vi "定时器更新溢出中断实验.vi"   [LabVIEW 2011]
uses:
  <vilib>/STM32_DriverVI_Interface_F4/Timer/TIMX Interrupt_F4.ctl
  <vilib>/STM32_DriverVI_Interface/Interrupt/PreemptionPriority_0.ctl
  <vilib>/STM32_DriverVI_Interface/Interrupt/SubPriority_0.ctl
  <vilib>/STM32_DriverVI_Interface_F4/Timer/TIM2_Int_Channel_F4.ctl
  <vilib>/STM32_DriverVI_Interface_F4/Timer/TIM2_Flag_F4.ctl
  <vilib>/STM32_DriverVI_Interface_F4/Timer/Reload Mode_F4.ctl
  <vilib>/STM32_DriverVI_Interface_F4/Timer/TIM2 Init_F4.vi
  <vilib>/STM32_DriverVI_Interface_F4/Timer/TIM Priority Set_0_F4.vi
  <vilib>/STM32_DriverVI_Interface_F4/Timer/TIM2 SW Interrupt_F4.vi
  <vilib>/STM32_DriverVI_Interface_F4/Timer/Clear_TIM2_Flag_F4.vi
  <vilib>/STM32_DriverVI_Interface_F4/Timer/TIM2 Int Permit_UnPermit_F4.vi
  <vilib>/STM32_DriverVI_Interface_F4/Timer/TIM2 Int Enable_Disable_F4.vi
  <vilib>/STM32_DriverVI_Interface_F4/Timer/TIM2 Update Interval_F4.vi
types:
  T1 = typedef "TIM2_Flag_F4.ctl" = enum8{"TIM2_Update(Overflow)", "TIM2_Channel_1", "TIM2_Channel_2", "TIM2_Channel_3", "TIM2_Channel_4", "TIM2_Reserved……", "TIM2_Trigger（Pulse）"}
  T2 = typedef "中断使能禁止.ctl" = enum8{"Disable", "Enable"}
  T3 = typedef "允许或禁止TIM中断_F4.ctl" = enum8{"禁止", "允许"}
  T4 = typedef "TIM2_Int_Channel_F4.ctl" = enum8{"TIM2_Update(Overflow)", "TIM2_Channel_1", "TIM2_Channel_2", "TIM2_Channel_3", "TIM2_Channel_4", "TIM2_Reserved……", "TIM2_Trigger（Pulse）"}
  T5 = typedef "SubPriority_0.ctl" = enum8{"Priority_0（High）", "Priority_1", "Priority_2", "Priority_3", "Priority_4", "Priority_5", "Priority_6", "Priority_7", "Priority_8", "Priority_9", "Priority_10", "Priority_11", "Priority_12", "Priority_13", "Priority_14", "Priority_15（Low）"}
  T6 = typedef "PreemptionPriority_0.ctl" = enum8{"Priority_0（Only）"}
  T7 = typedef "TIMX Interrupt_F4.ctl" = u8
  T8 = typedef "TIMX计数时钟频率_F4.ctl" = u16
  T9 = typedef "Reload Mode_F4.ctl" = enum8{"写入时立刻重载", "发生更新中断时重载"}
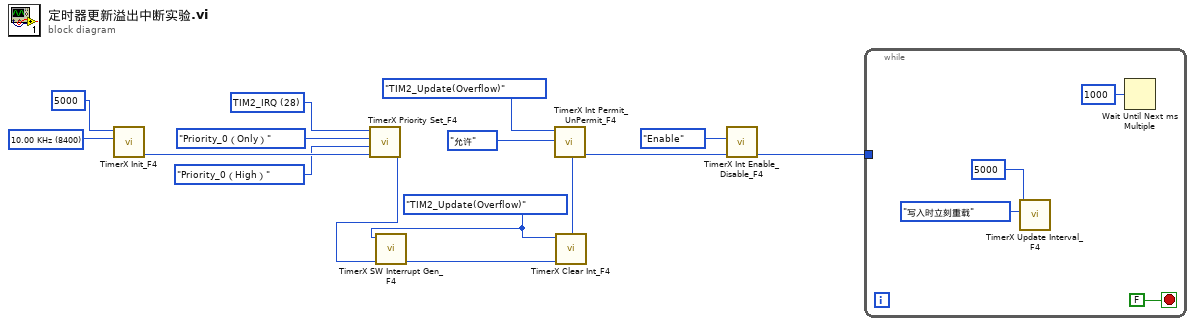
[diagram p0: block diagram]
diagram:
  w1 = TIM2_Flag_F4."TIM2_Update(Overflow)" ("TIM2_Flag")
  w13 = T7 28 items=["WWDG_IRQ"=0, "RTC_WKUP_IRQ"=3, "RTC_Alarm_IRQ"=41, "TIM1_BRK_TIM9_IRQ"=24, "TIM1_UP_TIM10_IRQ"=25, "TIM1_TRG_COM_TIM11_IRQ"=26, "TIM1_CC_IRQ"=27, "TIM2_IRQ"=28, "TIM3_IRQ"=29, "TIM4_IRQ"=30, "TIM5_IRQ"=50, "TIM6_IRQ"=54, "TIM7_IRQ"=55, "TIM8_BRK_TIM12_IRQ"=43, "TIM8_UP_TIM13_IRQ"=44, "TIM8_TRG_COM_TIM14_IRQ"=45, "TIM8_CC_IRQ"=46] ("IO 中断号设置")
  w14 = T8 8400 items=["84.00 MHz"=1, "42.00 MHz"=2, "28.00 MHz"=3, "21.00 MHz"=4, "12.000 MHz"=7, "7.000 MHz"=12, "4.000 MHz"=21, "1.000 MHz"=84, "-------------"=0, "500.0 KHz"=168, "250.0 KHz"=336, "100.0 KHz"=840, "50.00 KHz"=1680, "10.00 KHz"=8400] ("时钟预分频数")
  n1 = call-poly <vilib>:"TimerX Init_F4.vi"("时钟预分频数"=w14, "自动重装值"=u16 5000) -> ("err_out"=w12:u8)  [unwired: 9 in]
  n2 = call-poly <vilib>:"TimerX Priority Set_F4.vi"("err_in"=w12, "响应优先级"=SubPriority_0."Priority_0（High）", "抢占优先级"=PreemptionPriority_0."Priority_0（Only）", "TIM 中断号设置"=w13) -> ("err_out"=w3:u8)  [unwired: 6 in, 1 out]
  n3 = call-poly <vilib>:"TimerX SW Interrupt Gen_F4.vi"("err_in"=w3, "TIM2_Flag"=w1) -> ("err_out"=w4:u8)  [unwired: 9 in]
  n4 = call-poly <vilib>:"TimerX Clear Int_F4.vi"("err_in"=w4, "TIM2_Flag"=w1) -> ("err_out"=w2:u8)  [unwired: 9 in]
  n5 = call-poly <vilib>:"TimerX Int Permit_UnPermit_F4.vi"("err_in"=w2, "屏蔽或开启TIM2中断"=允许或禁止TIM中断_F4."允许", "TIM2_Int_Channel"=TIM2_Int_Channel_F4."TIM2_Update(Overflow)") -> ("err_out"=w11:u8)  [unwired: 8 in]
  n6 = call-poly <vilib>:"TimerX Int Enable_Disable_F4.vi"("err_in"=w11, "中断使能/关闭"=中断使能禁止."Enable") -> ("err_out"=w5:u8)  [unwired: 9 in]
  n7 = while {
    tunnel: w5 -> [_]
    stop <- FALSE stop-if-true
    n8 = call-poly <vilib>:"TimerX Update Interval_F4.vi"("中断时间间隔重载方式"=Reload_Mode_F4."写入时立刻重载", "TIM2 Interval Value[自动重装值]"=u16 5000) -> ()  [unwired: 9 in, 1 out]
    n9 = Wait Until Next ms Multiple(millisecond multiple=u32 1000 ("毫秒倍数")) -> ()  [unwired: 1 out]
  }
